vi "Forward Packet to Client.vi"(10 "Response":T1, 11 "Session in":refnum<class "Session.lvclass">) -> (0 "error out":errorcluster)   [LabVIEW 2013]
uses:
  Session.lvclass
  <vilib>/LabVIEW Open Source Project/MQTT Control Packets/Control Packets/ControlPacket/ControlPacket.lvclass
  Server/Connection/TCPConnection.lvclass
  Base Class/Response -- cluster.ctl
  Base Class/MQTT_Base.lvclass
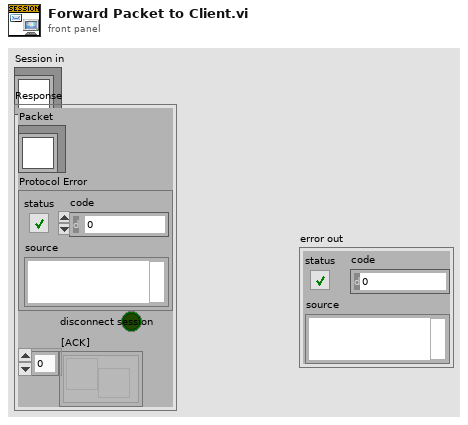
[diagram p1: front panel]
types:
  T1 = typedef "MQTT Base.lvlib/MQTT_Base.lvclass/Response -- cluster.ctl" = cluster{"Packet":refnum<class "ControlPacket.lvclass">, "Protocol Error":errorcluster, "disconnect session":bool, "[ACK]":refnum<notifier>[]}
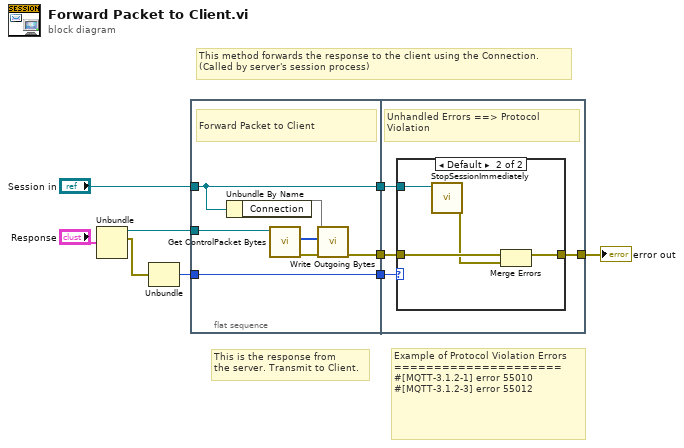
[diagram p0: block diagram]
diagram:
  # "This method forwards the response to the client using the Connection.\n(Called by server's session process)"
  # "This is the response from\nthe server. Transmit to Client."
  # "Example of Protocol Violation Errors\n=====================\n#[MQTT-3.1.2-1] error 55010\n#[MQTT-3.1.2-3] error 55012"
  n1 = Unbundle("Response") -> ("Packet"=w9:refnum<class "ControlPacket.lvclass">, "Protocol Error"=w5:errorcluster)  [unwired: 2 out]
  n2 = Unbundle(w5) -> ("code"=w2:i32)  [unwired: 2 out]
  n3 = flat-sequence {
    tunnel: w9 -> [w15]
    tunnel: "Session in" -> [w10]
    tunnel: [w13] -> w4
    tunnel: [w11] -> w3
    tunnel: w2 -> [w11]
    tunnel: [w10] -> w1
    tunnel: [w17] -> w7
    tunnel: w4 -> [w18]
    tunnel: w3 -> [w19]
    tunnel: w1 -> [w20]
    frame #0 {
      # "Forward Packet to Client"
      n4 = Unbundle By Name(w10) -> ("Connection"=w12)
      n5 = call <vilib>:"Get ControlPacket Bytes.vi"("ControlPacket"=w15) -> ("error out"=w14:errorcluster, "Bytes Stream"=w16:u8[])  [unwired: 7 in, 2 out]
      n6 = call "Write Outgoing Bytes.vi"("error in (no error)"=w14, "Bytes"=w16, "TCPConnection in"=w12) -> ("error out"=w13:errorcluster)  [unwired: 7 in, 1 out]
    }
    frame #1 {
      # "Unhandled Errors ==> Protocol Violation"
      n7 = case shown="Default" w19 {
        tunnel: w20 -> [_ w25]
        tunnel: w18 -> [w21 w24]
        tunnel: [w21 w22] -> w17
        frame 0 {
        }
        frame Default {
          n8 = call "StopSessionImmediately.vi"("Session in"=w25) -> ("error out"=w23:errorcluster)  [unwired: 9 in, 1 out]
          n9 = Merge Errors(w24, w23) -> (w22:errorcluster)
        }
      }
    }
  }
  "error out" <- w7
